vi "PowI8.vi"(4 "y":i8, 5 "x":i8) -> (1 "x^y":i8, 2 "Overflow?":bool)   [LabVIEW 2017, in "GPOverflow.lvlib"]
doc: "Computes <B>x</B> to the <B>y</B>'th power keeping track of numeric overflow.\n\n<B>Overflow?</B> will be True if positive or negative overflow occurred. The output will saturate in case of overflow.\n\nThis VI is inlined.\n\nSteen Schmidt\nGPower\n8/8 2013"
uses:
  GPOverflow.lvlib
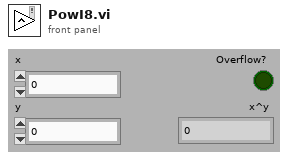
[diagram p1: front panel]
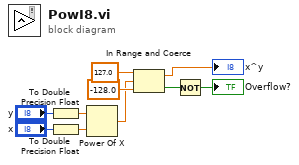
[diagram p0: block diagram]
diagram:
  n1 = To Double Precision Float(number="y") -> (double precision float=w8:dbl)
  n2 = To Double Precision Float(number="x") -> (double precision float=w7:dbl)
  n3 = Power Of X(1:w7, 2:w8) -> (0:w3:dbl)
  n4 = In Range and Coerce(upper limit=127.0, x=w3, lower limit=-128.0) -> (coerced(x)=→"x^y":dbl, In Range?=w4:bool)
  n5 = Not(x=w4) -> (.not. x?=→"Overflow?":bool)
